vi "fileObjectivesRegistrationSave.vi"(0 "xyz(opto)xyz(img)":dbl[][](array[numeric]), 1 "param":dbl[][](array[numeric]), 2 "normParam":dbl[](array[numeric]), 3 "denormParam":dbl[](array[numeric]), 4 "z(opto)z(img)":dbl[][](array[numeric])) -> ()   [LabVIEW 2017]
uses:
  globalUtilities.vi
  <vilib>/Utility/file.llb/Write Delimited Spreadsheet (DBL).vi
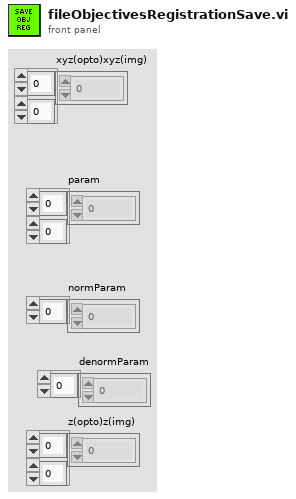
[diagram p1: front panel]
types:
  T1 = enum16{"open", "replace", "create", "open or create", "replace or create", "replace or create with confirmation"}
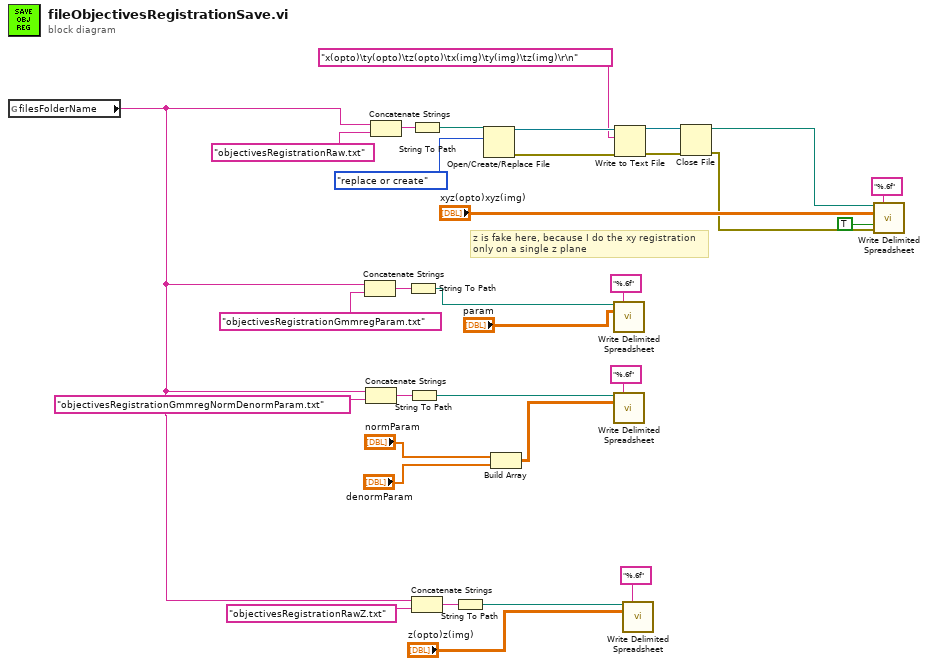
[diagram p0: block diagram]
diagram:
  # "z is fake here, because I do the xy registration\nonly on a single z plane"
  n1 = global read "globalUtilities.vi" "filesFolderName"() -> (w3:string)
  n2 = Concatenate Strings(w3, "objectivesRegistrationGmmregParam.txt" ("string")) -> (w16:string)
  n3 = Concatenate Strings(w3, "objectivesRegistrationGmmregNormDenormParam.txt" ("string")) -> (w9:string)
  n4 = Concatenate Strings(w3, "objectivesRegistrationRaw.txt" ("string")) -> (w22:string)
  n5 = String To Path(string=w16) -> (path=w15:path)
  n6 = String To Path(string=w9) -> (path=w8:path)
  n7 = String To Path(string=w22) -> (path=w21:path)
  n8 = Concatenate Strings(w3, "objectivesRegistrationRawZ.txt" ("string")) -> (w5:string)
  n9 = String To Path(string=w5) -> (path=w2:path)
  n10 = Open/Create/Replace File(file path (use dialog)=w21, operation (0:open)=T1."replace or create") -> (refnum out=w29:refnum<file>, error out=w26:errorcluster)  [unwired: 4 in, 1 out]
  n11 = Build Array("normParam", "denormParam") -> (w7:dbl[][])
  n12 = call-poly <vilib>:"Write Delimited Spreadsheet.vi"("file path (dialog if empty)"=w15, "format (%.3f)"="%.6f", "2D data"="param") -> ()  [unwired: 11 in, 2 out]
  n13 = call-poly <vilib>:"Write Delimited Spreadsheet.vi"("file path (dialog if empty)"=w8, "format (%.3f)"="%.6f", "2D data"=w7) -> ()  [unwired: 11 in, 2 out]
  n14 = Write to Text File(file (use dialog)=w29, text="x(opto)\ty(opto)\tz(opto)\tx(img)\ty(img)\tz(img)\r\n", error in=w26) -> (refnum out=w27:refnum<file>, error out=w25:errorcluster)  [unwired: 1 in, 1 out]
  n15 = call-poly <vilib>:"Write Delimited Spreadsheet.vi"("file path (dialog if empty)"=w2, "format (%.3f)"="%.6f", "2D data"="z(opto)z(img)") -> ()  [unwired: 11 in, 2 out]
  n16 = Close File(refnum=w27, error in=w25) -> (path=w19:path, error out=w24:errorcluster)
  n17 = call-poly <vilib>:"Write Delimited Spreadsheet.vi"("file path (dialog if empty)"=w19, "format (%.3f)"="%.6f", "2D data"="xyz(opto)xyz(img)", "append to file? (new file:F)"=TRUE, "error in (no error)"=w24) -> ()  [unwired: 9 in, 2 out]
